vi "ISX3_Cmd_SetExtPortChannel.vi"(1 "WS-Port":u8, 2 "W-Port":u8, 3 "R-Port":u8, 4 "C-Port":u8) -> (0 "set channel Cmd":u8[](array[numeric]))   [LabVIEW 2012, in "Sciospec ISX3 Impedance Analyzer.lvlib"]
uses:
  Sciospec ISX3 Impedance Analyzer.lvlib
panel:
  # "This VI generates the command to set the EextensionPort channel\nfor the next measurement."
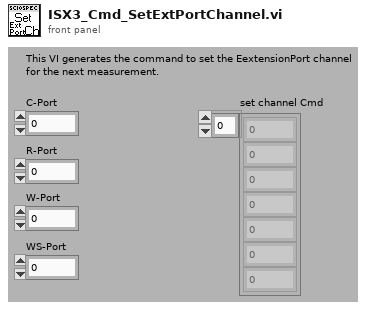
[diagram p1: front panel]
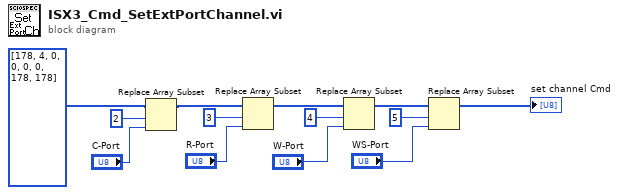
[diagram p0: block diagram]
diagram:
  n1 = Replace Array Subset(array=u8[] [178, 4, 0, 0, 0, 0, 178, 178], new element="C-Port", index=2) -> (w11:u8[])
  n2 = Replace Array Subset(array=w11, new element="R-Port", index=3) -> (w5:u8[])
  n3 = Replace Array Subset(array=w5, new element="W-Port", index=4) -> (w2:u8[])
  n4 = Replace Array Subset(array=w2, new element="WS-Port", index=5) -> (→"set channel Cmd":u8[])
